vi "Execute Publication Policy.vi"(7 "Default PublicationPolicy":refnum<class "IPublicationPolicy.lvclass">, 9 "Last Publish Time":timestamp, 10 "Last Published Value":variant, 11 "PublishRequest":refnum<class "PublishRequest.lvclass">) -> (0 "error out (Reject Publication)":errorcluster, 1 "Publication Time":timestamp, 2 "Value to Publish":variant)   [LabVIEW 2017, in "IMediator.lvlib" / "PublishRequest.lvclass"]
doc: "This method decides whether or not to send or otherwise handle the new data value. The policy is set and maintained by the subscriber. The Topic Actor knows no policy details, it just passes the new value in. If there is a failure inside this method, the Topic Actor must assume the listener is no longer valid (dead/unrecoverable) and should delete it from the Subscriber list.\n\n<License>\nCopyright © 2017 Composed Systems, LLC | All rights reserved\nwww.composed.io\n\nAuthor: Ethan Stern <ethan.stern@composed.io>\n\nThis software is provided \"AS IS\" WITHOUT WARRANTIES, either express or implied, AND IS FOR EDUCATIONAL PURPOSES ONLY.\n</License>"
uses:
  PublishRequest.lvclass
  IPublicationPolicy/IPublicationPolicy.lvclass
  PublishRequest.lvclass/PublishRequest.ctl
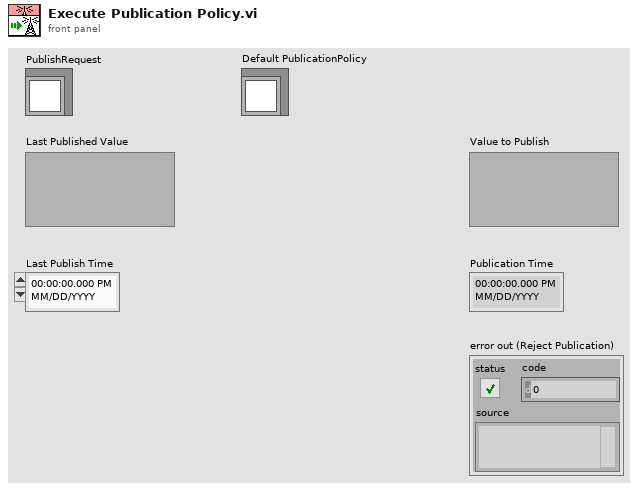
[diagram p1: front panel]
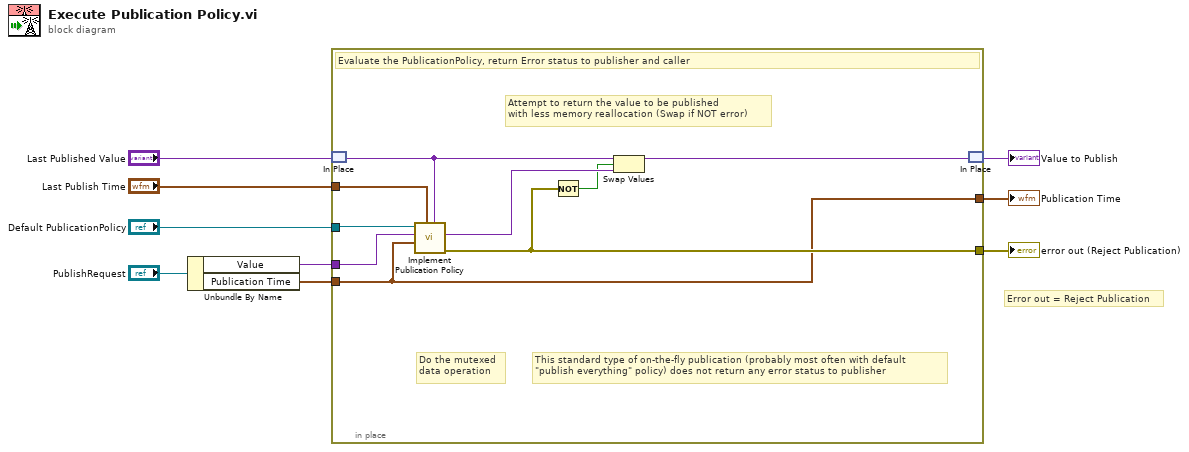
[diagram p0: block diagram]
diagram:
  # "Error out = Reject Publication"
  n1 = Unbundle By Name("PublishRequest") -> ("Value"=w3:variant, "Publication Time"=w2:timestamp)
  n2 = in-place {
    in-place-border: [w11] -> w8
    in-place-border: "Default PublicationPolicy" -> [w15]
    in-place-border: w3 -> [w14]
    in-place-border: w2 -> [w10]
    in-place-border: "Last Publish Time" -> [w12]
    in-place-border: [w10] -> w1
    # "This standard type of on-the-fly publication (probably most often with default\n\"publish everything\" policy) does not return any error status to publisher"
    # "Do the mutexed\ndata operation"
    # "Attempt to return the value to be published\nwith less memory reallocation (Swap if NOT error)"
    # "Evaluate the PublicationPolicy, return Error status to publisher and caller"
    n3 = in-place-match #1("Last Published Value") -> (w13:variant)
    n4 = call-dynamic "Implement Publication Policy.vi"("Last Published Value"=w13, "Last Published Time"=w12, "New Value Time"=w10, "New Value"=w14, "PublicationPolicy"=w15) -> ("error out (Reject Publication)"=w11:errorcluster, "Value to Publish"=w17:variant)  [unwired: 5 in]
    n5 = Not(x=w11) -> (.not. x?=w16:bool)
    n6 = Swap Values(12:w13, 13:w16, 14:w17) -> (1:w18:variant)  [unwired: 1 out]
    n7 = in-place-match #1(w18) -> (→"Value to Publish":variant)
  }
  "error out (Reject Publication)" <- w8
  "Publication Time" <- w1
